vi "Periodic Tasks.vi"() -> ()   [LabVIEW 2011]
doc: "This VI runs in parallel to other tasks. It can contain as many user-defined periodic loops as you need. These can carry out PID or other sorts of timed response."
uses:
  <vilib>/Rock Robotics/SystemInterfaces/Utilities/FPGA_UtilitiesLED State.ctl
  <vilib>/Rock Robotics/SystemInterfaces/Utilities/FPGA_UtilitiesLED Source.ctl
  Robot Global Data.vi
  <vilib>/Rock Robotics/WPI/Relay/WPI_RelayValue.ctl
panel:
  in  "Reset Ball":bool
  in  "Home Speed":dbl=0.4
  out "Auton Recording":bool
  in  "Turn on Record":bool
  in  "Auton Array":dbl[][](array[numeric])
  out "Ramp ACT Pot":dbl
  out "Right Rate":dbl
  out "Right Direction":bool
  out "Right Distance":dbl
  out "Shooter Encoder Distance":dbl
  out "Shooter Direction":bool
  out "Shooter Encoder Rate":dbl
  out "Left Rate":dbl
  out "Gyro Rate":dbl
  out "Gyro Angle":dbl
  out "Left Direction":bool
  out "Left Distance":dbl
  # "Auton Recording"
  # "Sensor Feedback"
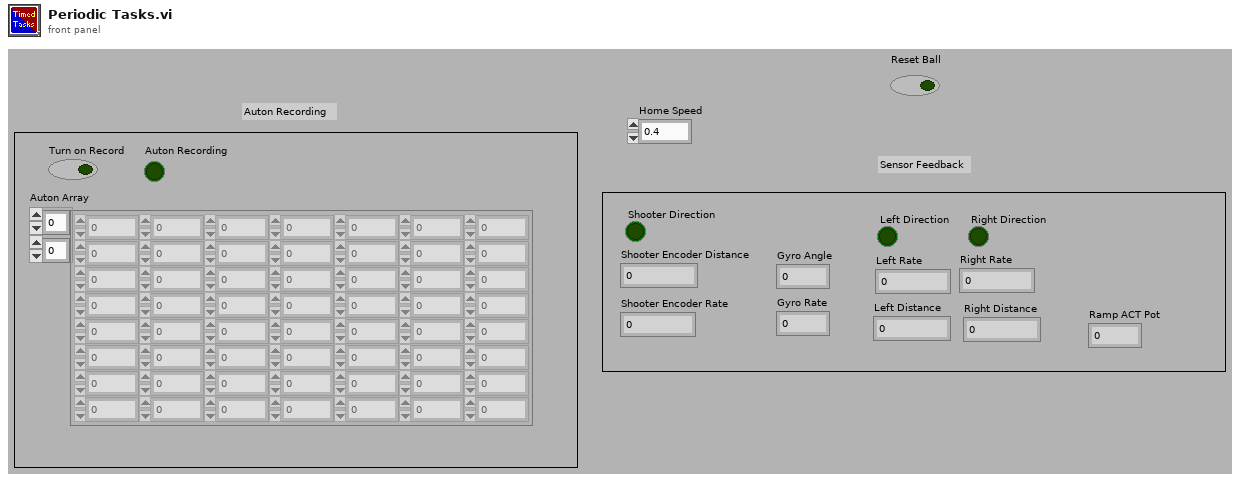
[diagram p1: front panel]
types:
  T1 = typedef "WPI_RelayValue.ctl" = enum16{"Off", "On", "Forward", "Reverse"}
  T2 = typedef "WPI_AnalogChannelDevRef.ctl" = cluster{"DevStatus":errorcluster, "Analog Module":T3, "Analog Channel":T4}
  T3 = typedef "FPGA_TypedefAnalogModule.ctl" = enum16{"Analog Module 1", "Analog Module 2"}
  T4 = typedef "FPGA_AIChannel.ctl" = enum8{"AI 1", "AI 2", "AI 3", "AI 4", "AI 5", "AI 6", "AI 7", "AI 8", "Invalid"}
  T5 = typedef "WPI_EncoderDevRef.ctl" = cluster{"DevStatus":errorcluster, "EncoderIndex":T6, "CounterIndex":T7, "DistancePerCount":dbl, "Decoding Type":T8}
  T6 = typedef "FPGA_EncoderIdx.ctl" = enum8{"Enc 0", "Enc 1", "Enc 2", "Enc 3", "Invalid"}
  T7 = typedef "FPGA_CounterCtrSystemIndex.ctl" = enum8{"Ctr 0", "Ctr 1", "Ctr 2", "Ctr 3", "Ctr 4", "Ctr 5", "Ctr 6", "Ctr 7", "Invalid"}
  T8 = typedef "WPI_EncoderType.ctl" = enum16{"1x", "2x", "4x"}
  T9 = typedef "WPI_GyroDevRef.ctl" = cluster{"DevStatus":errorcluster, "Analog Module":T3, "Analog Channel":T4, "Offset":dbl, "Gain (VoltsPerDegree/Second)":dbl}
  T10 = typedef "WPI_RelayDevRef.ctl" = cluster{"DevStatus":errorcluster, "Relay Channel":T11, "Digital Module":T12, "Relay Direction":T13}
  T11 = typedef "FPGA_DIORelayChannel.ctl" = enum8{"Relay 1", "Relay 2", "Relay 3", "Relay 4", "Relay 5", "Relay 6", "Relay 7", "Relay 8", "Invalid"}
  T12 = typedef "FPGA_TypedefDigitalModule.ctl" = enum16{"Digital Module 1", "Digital Module 2"}
  T13 = typedef "WPI_RelayDirection.ctl" = enum16{"Both directions", "Forward only", "Reverse only"}
  T14 = typedef "FPGA_UtilitiesLED State.ctl" = enum16{"Off", "On", "Toggle"}
  T15 = typedef "FPGA_UtilitiesLED Source.ctl" = enum16{"User LED", "FPGA LED"}
  T16 = cluster{"Left Drive Output":dbl, "Right Drive Output":dbl, "Ramp Actuator Output":dbl, "Harvester Output":dbl, "Conveyer Output":dbl, "Turret Rotation":dbl, "Shooter Output":dbl}
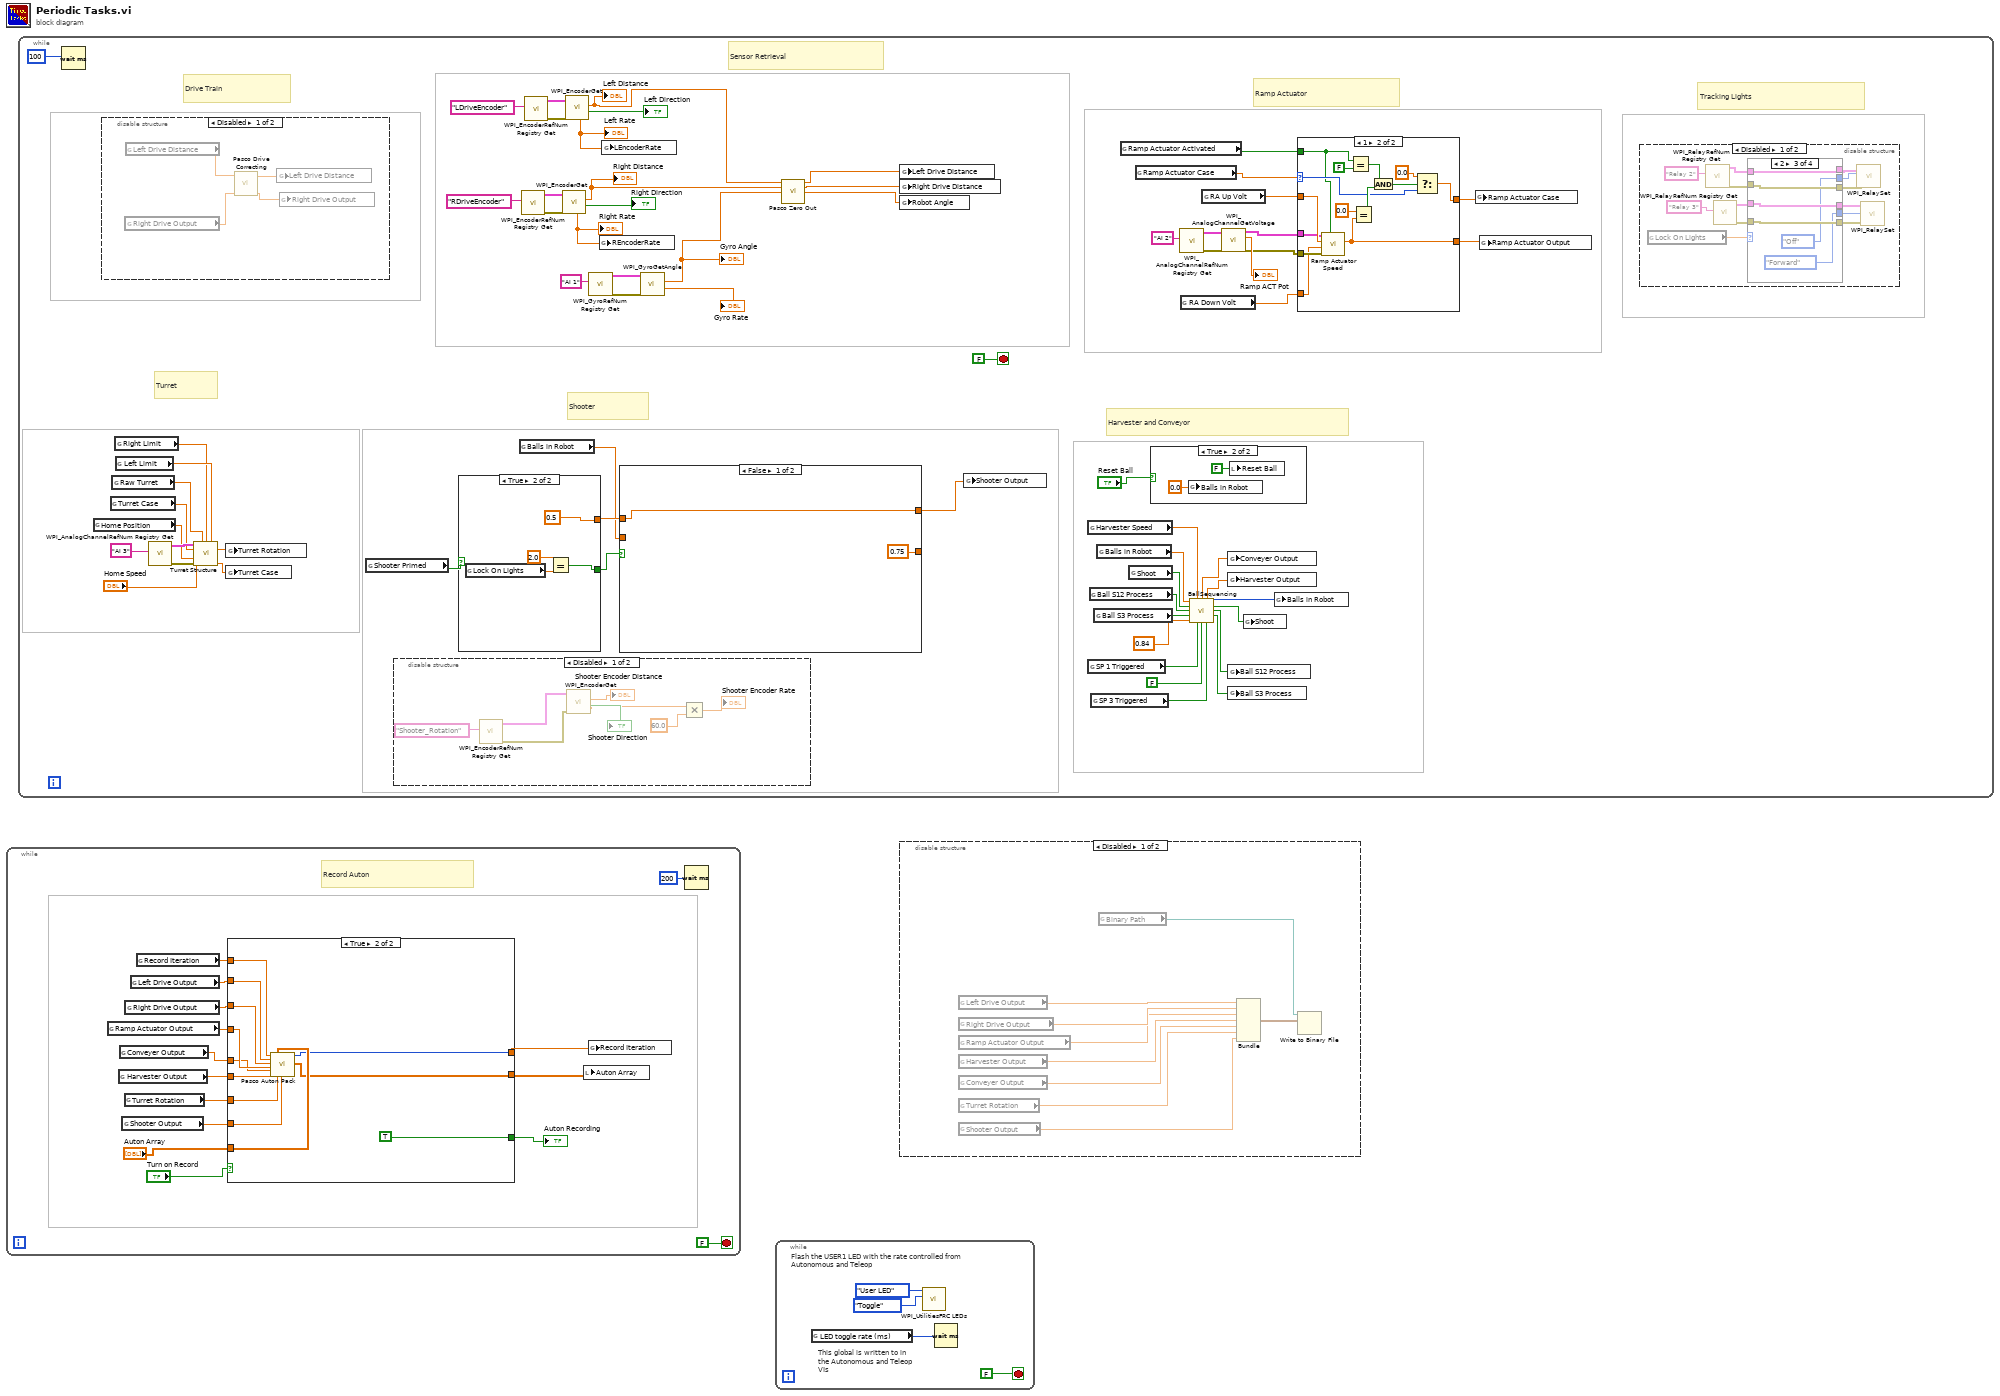
[diagram p0: block diagram]
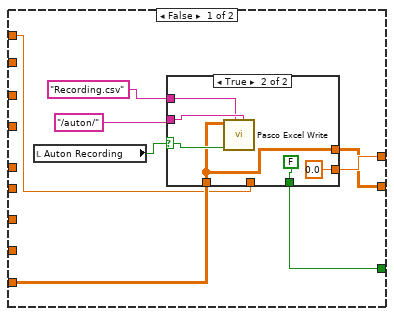
[diagram p2: hidden frame]
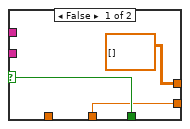
[diagram p3: hidden frame]
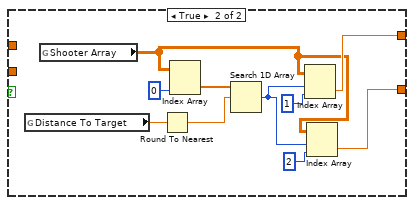
[diagram p5: hidden frame]
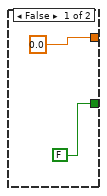
[diagram p6: hidden frame]
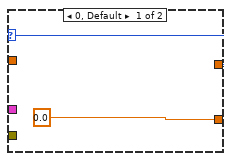
[diagram p8: hidden frame]
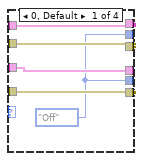
[diagram p9: hidden frame]
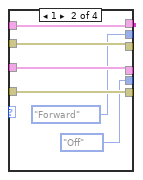
[diagram p10: hidden frame]
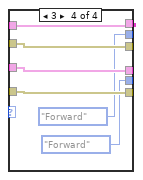
[diagram p11: hidden frame]
diagram:
  n1 = while {
    stop <- FALSE stop-if-true
    # "Record Auton"
    n2 = global read "Robot Global Data.vi" "Ramp Actuator Output"() -> (w5:dbl)
    n3 = global read "Robot Global Data.vi" "Harvester Output"() -> (w7:dbl)
    n4 = global read "Robot Global Data.vi" "Conveyer Output"() -> (w6:dbl)
    n5 = global read "Robot Global Data.vi" "Shooter Output"() -> (w9:dbl)
    n6 = global read "Robot Global Data.vi" "Turret Rotation"() -> (w8:dbl)
    n7 = global read "Robot Global Data.vi" "Right Drive Output"() -> (w4:dbl)
    n8 = global read "Robot Global Data.vi" "Left Drive Output"() -> (w3:dbl)
    n9 = global read "Robot Global Data.vi" "Record Iteration"() -> (w2:dbl)
    n10 = case shown="True" "Turn on Record" {
      tunnel: w2 -> [w19 w44]
      tunnel: w3 -> [_ w43]
      tunnel: w4 -> [_ w42]
      tunnel: w5 -> [_ w41]
      tunnel: w6 -> [_ w40]
      tunnel: w7 -> [_ w39]
      tunnel: w8 -> [_ w38]
      tunnel: w9 -> [_ w37]
      tunnel: "Auton Array" -> [w20 w36]
      tunnel: [w16 w35] -> w12
      tunnel: [w17 w34] -> w13
      tunnel: [w18 TRUE] -> w14
      frame False {
        n11 = local read "Auton Recording"() -> (w21:bool)
        n12 = case shown="True" w21 {
          selector: w21 -> [w26 w31]
          tunnel: [w26 FALSE] -> w18
          tunnel: "/auton/" ("File Name") -> [_ w30]
          tunnel: "Recording.csv" ("Folder Location") -> [_ w29]
          tunnel: [w25 0.0 ("Record Iteration")] -> w17
          tunnel: w19 -> [w25 _]
          tunnel: w20 -> [_ w27]
          tunnel: [dbl[][] [] ("Auton Array") w27] -> w16
          frame False {
          }
          frame True {
            n13 = call "Pasco Excel Write.vi"("Folder Location"=w30, "File Name"=w29, "WriteToExcel"=w31, "2D data"=w27) -> ()  [unwired: 7 in, 1 out]
          }
        }
      }
      frame True {
        n14 = call "Pasco Auton Pack.vi"("Iterations"=w44, "Left Drive"=w43, "Right Drive"=w42, "RAMP ACT"=w41, "Conveyor"=w40, "Harvestor"=w39, "Auton Array"=w36, "Turret"=w38, "Shooter"=w37) -> ("Iteration Output"=w34:i32, "output array"=w35:dbl[][])  [unwired: 9 in]
      }
    }
    "Auton Recording" <- w14
    n15 = local write "Auton Array"(w12) -> ()
    n16 = global write "Robot Global Data.vi" "Record Iteration"(w13) -> ()
    n17 = Wait (ms)(milliseconds to wait=u32 200) -> ()  [unwired: 1 out]
  }
  n18 = while {
    stop <- FALSE stop-if-true
    # "Tracking Lights"
    # "Harvester and Conveyor"
    # "Shooter"
    # "Sensor Retrieval"
    # "Turret"
    # "Drive Train"
    # "Ramp Actuator"
    n19 = Wait (ms)(milliseconds to wait=u32 100) -> ()  [unwired: 1 out]
    n20 = global read "Robot Global Data.vi" "Home Position"() -> (w104:dbl)
    n21 = disable-structure shown="Disabled" {
      frame Disabled {
        n22 = global read "Robot Global Data.vi" "Right Drive Output"() -> (w185:dbl)
        n23 = global read "Robot Global Data.vi" "Left Drive Distance"() -> (w186:dbl)
        n24 = call "Pasco Drive Correcting.vi"("RightDriveOutput"=w185, "LeftDriveOutput"=w186) -> ("RightDriveOutput"=w183:dbl, "LeftDriveOutput"=w184:dbl)  [unwired: 8 in]
        n25 = global write "Robot Global Data.vi" "Left Drive Distance"(w184) -> ()
        n26 = global write "Robot Global Data.vi" "Right Drive Output"(w183) -> ()
      }
      frame Enabled {
      }
    }
    n27 = global read "Robot Global Data.vi" "Turret Case"() -> (w105:dbl)
    n28 = global read "Robot Global Data.vi" "Raw Turret"() -> (w103:dbl)
    n29 = global read "Robot Global Data.vi" "Right Limit"() -> (w86:dbl)
    n30 = global read "Robot Global Data.vi" "Left Limit"() -> (w87:dbl)
    n31 = call <vilib>:"WPI_AnalogChannelRefNum Registry Get.vi"("refnum name"="AI 3") -> ("error out"=w106:errorcluster, "AIDeviceRef"=w107:T2)  [unwired: 9 in]
    n32 = call "Turret Structure.vi"("AIDeviceRef"=w107, "Raw Turret"=w103, "upper limit"=w86, "lower limit"=w87, "Turret Case"=w105, "Home Speed"="Home Speed", "Home postion"=w104, "error in (no error)"=w106) -> ("Turret Output"=w102:dbl, "Turret Case Output"=w101:dbl)  [unwired: 6 in]
    n33 = global write "Robot Global Data.vi" "Turret Rotation"(w102) -> ()
    n34 = global write "Robot Global Data.vi" "Turret Case"(w101) -> ()
    n35 = global read "Robot Global Data.vi" "Shooter Primed"() -> (w73:bool)
    n36 = disable-structure shown="Disabled" {
      frame Disabled {
        n37 = call <vilib>:"WPI_EncoderRefNum Registry Get.vi"("refnum name"="Shooter_Rotation") -> ("error out"=w187:errorcluster, "EncoderDevRef"=w188:T5)  [unwired: 9 in]
        n38 = call <vilib>:"WPI_EncoderGet.vi"("error in (no error)"=w187, "EncoderDevRef"=w188) -> ("Direction"=→"Shooter Direction":bool, "Distance"=→"Shooter Encoder Distance":dbl, "Rate"=w191:dbl)  [unwired: 4 in, 3 out]
        n39 = Multiply(x=w191, y=60.0) -> (x*y=→"Shooter Encoder Rate":dbl)
      }
      frame Enabled {
      }
    }
    n40 = case shown="True" w73 {
      tunnel: [FALSE ("Shooter Primed") w125] -> w72
      tunnel: [0.0 0.5] -> w70
      frame False {
      }
      frame True {
        n41 = global read "Robot Global Data.vi" "Lock On Lights"() -> (w127:dbl)
        n42 = Equal?(x=2.0, y=w127) -> (x = y?=w125:bool)
      }
    }
    n43 = global read "Robot Global Data.vi" "Balls in Robot"() -> (w69:dbl)
    n44 = call <vilib>:"WPI_EncoderRefNum Registry Get.vi"("refnum name"="RDriveEncoder") -> ("error out"=w54:errorcluster, "EncoderDevRef"=w53:T5)  [unwired: 9 in]
    n45 = call <vilib>:"WPI_EncoderRefNum Registry Get.vi"("refnum name"="LDriveEncoder") -> ("error out"=w59:errorcluster, "EncoderDevRef"=w58:T5)  [unwired: 9 in]
    n46 = call <vilib>:"WPI_EncoderGet.vi"("error in (no error)"=w54, "EncoderDevRef"=w53) -> ("Direction"=→"Right Direction":bool, "Distance"=w50:dbl, "Rate"=w51:dbl)  [unwired: 4 in, 3 out]
    "Right Distance" <- w50
    "Right Rate" <- w51
    n47 = call <vilib>:"WPI_EncoderGet.vi"("error in (no error)"=w59, "EncoderDevRef"=w58) -> ("Direction"=→"Left Direction":bool, "Distance"=w49:dbl, "Rate"=w56:dbl)  [unwired: 4 in, 3 out]
    "Left Distance" <- w49
    "Left Rate" <- w56
    n48 = call <vilib>:"WPI_GyroRefNum Registry Get.vi"("refnum name"="AI 1") -> ("error out"=w66:errorcluster, "GyroDevRef"=w67:T9)  [unwired: 9 in]
    n49 = global write "Robot Global Data.vi" "REncoderRate"(w51) -> ()
    n50 = global write "Robot Global Data.vi" "LEncoderRate"(w56) -> ()
    n51 = case shown="False" w72 {
      tunnel: [w112 w122] -> w71
      tunnel: w70 -> [w112 _]
      tunnel: w69 -> [_ _]
      tunnel: [0.75 w121] -> _
      frame False {
      }
      frame True {
        n52 = global read "Robot Global Data.vi" "Distance To Target"() -> (w118:dbl)
        n53 = global read "Robot Global Data.vi" "Shooter Array"() -> (w113:dbl[][])
        n54 = Round To Nearest(number=w118) -> (nearest integer value=w117:dbl)
        n55 = Index Array(array=w113, index (col)=0 ("disabled index (col)")) -> (element=w116:dbl[])  [unwired: 1 in]
        n56 = Search 1D Array(1D array=w116, element=w117) -> (index of element=w114:i32)  [unwired: 1 in]
        n57 = Index Array(array=w113, index (row)=w114, index (col)=1 ("disabled index (col)")) -> (element=w122:dbl)
        n58 = Index Array(array=w113, index (row)=w114, index (col)=2 ("disabled index (col)")) -> (element=w121:dbl)
      }
    }
    n59 = call <vilib>:"WPI_GyroGetAngle.vi"("error in (no error)"=w66, "GyroDevRef"=w67) -> ("Angular Rate"=→"Gyro Rate":dbl, "Angle"=w48:dbl)  [unwired: 6 in, 2 out]
    "Gyro Angle" <- w48
    n60 = call "Pasco Zero Out.vi"("LDrive Distance"=w49, "RDrive Distance"=w50, "Gyro Heading"=w48) -> ("LDrive Distance"=w46:dbl, "RDrive Distance"=w47:dbl, "Gyro Heading"=w45:dbl)  [unwired: 10 in]
    n61 = global write "Robot Global Data.vi" "Left Drive Distance"(w46) -> ()
    n62 = global write "Robot Global Data.vi" "Right Drive Distance"(w47) -> ()
    n63 = global write "Robot Global Data.vi" "Robot Angle"(w45) -> ()
    n64 = global write "Robot Global Data.vi" "Shooter Output"(w71) -> ()
    n65 = global read "Robot Global Data.vi" "Harvester Speed"() -> (w68:dbl)
    n66 = global read "Robot Global Data.vi" "SP 1 Triggered"() -> (w77:bool)
    n67 = global read "Robot Global Data.vi" "Ball S12 Process"() -> (w79:bool)
    n68 = global read "Robot Global Data.vi" "SP 3 Triggered"() -> (w76:bool)
    n69 = global read "Robot Global Data.vi" "Ball S3 Process"() -> (w78:bool)
    n70 = global read "Robot Global Data.vi" "Balls in Robot"() -> (w81:dbl)
    n71 = global read "Robot Global Data.vi" "Ramp Actuator Activated"() -> (w94:bool)
    n72 = global read "Robot Global Data.vi" "Shoot"() -> (w80:bool)
    n73 = global read "Robot Global Data.vi" "Ramp Actuator Case"() -> (w96:dbl)
    n74 = case shown="True" "Reset Ball" {
      frame False {
      }
      frame True {
        n75 = global write "Robot Global Data.vi" "Balls in Robot"(0.0 ("Balls in Robot")) -> ()
        n76 = local write "Reset Ball"(FALSE ("Reset Ball")) -> ()
      }
    }
    n77 = call <vilib>:"WPI_AnalogChannelRefNum Registry Get.vi"("refnum name"="AI 2") -> ("error out"=w92:errorcluster, "AIDeviceRef"=w93:T2)  [unwired: 9 in]
    n78 = global read "Robot Global Data.vi" "RA Down Volt"() -> (w99:dbl)
    n79 = call "BallSequencing.vi"("Balls In Robot"=w81, "Speed of Harvester"=w68, "Shoot"=w80, "Ball S12 Process"=w79, "Ball S3 Process"=w78, "Speed of Conveyor"=0.84, "SP 1 Triggered"=w77, "SP 2 Triggered"=FALSE, "SP 3 Triggered"=w76) -> ("Conveyer Output"=w82:dbl, "Harvester Output"=w83:dbl, "Balls In Robot Output"=w62:i32, "Shoot Output"=w61:bool, "Ball S12 Process Output"=w85:bool, "Ball S3 Process Output"=w84:bool)  [unwired: 1 in]
    n80 = global read "Robot Global Data.vi" "RA Up Volt"() -> (w98:dbl)
    n81 = call <vilib>:"WPI_AnalogChannelGetVoltage.vi"("error in (no error)"=w92, "AIDeviceRef"=w93) -> ("error out"=w89:errorcluster, "Voltage"=→"Ramp ACT Pot":dbl, "AIDeviceRef"=w90:T2)  [unwired: 7 in]
    n82 = global write "Robot Global Data.vi" "Conveyer Output"(w82) -> ()
    n83 = global write "Robot Global Data.vi" "Harvester Output"(w83) -> ()
    n84 = global write "Robot Global Data.vi" "Ball S12 Process"(w85) -> ()
    n85 = global write "Robot Global Data.vi" "Ball S3 Process"(w84) -> ()
    n86 = global write "Robot Global Data.vi" "Shoot"(w61) -> ()
    n87 = global write "Robot Global Data.vi" "Balls in Robot"(w62) -> ()
    n88 = case shown="1" w96 {
      selector: w96 -> [w131 w136]
      tunnel: w89 -> [_ w146]
      tunnel: w99 -> [_ w145]
      tunnel: w98 -> [_ w144]
      tunnel: [0.0 ("Ramp Actuator Ouput") w135] -> w97
      tunnel: w94 -> [_ w134]
      tunnel: [w131 w137] -> w95
      tunnel: w90 -> [_ w133]
      frame 0, Default {
      }
      frame 1 {
        n89 = call "Ramp Actuator Speed.vi"("Up to Down"=w134, "error in (no error)"=w146, "RA Down Volt"=w145, "RA Up Volt"=w144, "AIDeviceRef"=w133) -> ("Ramp Actuator Ouput"=w135:dbl)  [unwired: 6 in]
        n90 = Equal?(x=w134, y=FALSE) -> (x = y?=w141:bool)
        n91 = Equal?(x=0.0, y=w135) -> (x = y?=w142:bool)
        n92 = And(x=w141, y=w142) -> (x .and. y?=w139:bool)
        n93 = Select(t=0.0, s=w139, f=w136) -> (s? t:f=w137:dbl)
      }
    }
    n94 = global write "Robot Global Data.vi" "Ramp Actuator Case"(w95) -> ()
    n95 = global write "Robot Global Data.vi" "Ramp Actuator Output"(w97) -> ()
    n96 = disable-structure shown="Disabled" {
      frame Disabled {
        n97 = global read "Robot Global Data.vi" "Lock On Lights"() -> (w147:dbl)
        n98 = call <vilib>:"WPI_RelayRefNum Registry Get.vi"("refnum name"="Relay 2") -> ("error out"=w154:errorcluster, "RelayDevRef"=w156:T10)  [unwired: 9 in]
        n99 = call <vilib>:"WPI_RelayRefNum Registry Get.vi"("refnum name"="Relay 3") -> ("error out"=w151:errorcluster, "RelayDevRef"=w152:T10)  [unwired: 9 in]
        n100 = case shown="2" w147 {
          tunnel: [w164 w170 w176 w182] -> w157
          tunnel: w156 -> [w164 w170 w176 w182]
          tunnel: [w163 w169 w175 w181] -> w155
          tunnel: w154 -> [w163 w169 w175 w181]
          tunnel: [w162 w168 w174 w180] -> w153
          tunnel: w152 -> [w162 w168 w174 w180]
          tunnel: w151 -> [w161 w167 w173 w179]
          tunnel: [w161 w167 w173 w179] -> w150
          tunnel: [w160 WPI_RelayValue."Forward" ("RelayValue") WPI_RelayValue."Off" ("RelayValue") WPI_RelayValue."Forward" ("RelayValue")] -> w149
          tunnel: [w160 WPI_RelayValue."Off" ("RelayValue") WPI_RelayValue."Forward" ("RelayValue") WPI_RelayValue."Forward" ("RelayValue")] -> w148
          frame 0, Default {
            w160 = WPI_RelayValue."Off" ("RelayValue")
          }
          frame 1 {
          }
          frame 2 {
          }
          frame 3 {
          }
        }
        n101 = call <vilib>:"WPI_RelaySet.vi"("error in (no error)"=w155, "RelayValue"=w149, "RelayDevRef"=w157) -> ()  [unwired: 7 in, 2 out]
        n102 = call <vilib>:"WPI_RelaySet.vi"("error in (no error)"=w150, "RelayValue"=w148, "RelayDevRef"=w153) -> ()  [unwired: 7 in, 2 out]
      }
      frame Enabled {
      }
    }
  }
  n103 = while {
    stop <- FALSE stop-if-true
    # "This global is written to in the Autonomous and Teleop VIs"
    # "Flash the USER1 LED with the rate controlled from Autonomous and Teleop"
    n104 = global read "Robot Global Data.vi" "LED toggle rate (ms)"() -> (w195:u32)
    n105 = call <vilib>:"WPI_UtilitiesFRC LEDs.vi"("State"=FPGA_UtilitiesLED_State."Toggle", "LED Type"=FPGA_UtilitiesLED_Source."User LED") -> ()  [unwired: 1 in, 9 out]
    n106 = Wait (ms)(milliseconds to wait=w195) -> ()  [unwired: 1 out]
  }
  n107 = disable-structure shown="Disabled" {
    frame Disabled {
      n108 = global read "Robot Global Data.vi" "Left Drive Output"() -> (w207:dbl)
      n109 = global read "Robot Global Data.vi" "Right Drive Output"() -> (w206:dbl)
      n110 = global read "Robot Global Data.vi" "Ramp Actuator Output"() -> (w205:dbl)
      n111 = global read "Robot Global Data.vi" "Harvester Output"() -> (w204:dbl)
      n112 = global read "Robot Global Data.vi" "Conveyer Output"() -> (w203:dbl)
      n113 = global read "Robot Global Data.vi" "Turret Rotation"() -> (w202:dbl)
      n114 = global read "Robot Global Data.vi" "Shooter Output"() -> (w201:dbl)
      n115 = global read "Robot Global Data.vi" "Binary Path"() -> (w199:path)
      n116 = Bundle("Left Drive Output"=w207, "Right Drive Output"=w206, "Ramp Actuator Output"=w205, "Harvester Output"=w204, "Conveyer Output"=w203, "Turret Rotation"=w202, "Shooter Output"=w201) -> (w200:T16)  [unwired: 1 in]
      n117 = Write to Binary File(file (use dialog)=w199, data=w200) -> ()  [unwired: 4 in, 3 out]
    }
    frame Enabled {
    }
  }
